vi "Remove Subscriber by Name.vi"(8 "error in (no error)":errorcluster, 10 "Topic Name":string, 11 "Subscriber Look Up Table in":refnum<class "Subscriber Look Up Table.lvclass">) -> (0 "error out":errorcluster, 2 "Found?":bool, 3 "Subscriber Look Up Table out":refnum<class "Subscriber Look Up Table.lvclass">)   [LabVIEW 2016, in "Stream Mediator.lvlib" / "Subscriber Look Up Table.lvclass"]
doc: "--\nCopyright © 2017 Composed SystemsI All rights reserved.\n\nAuthor: Jon McBee <jon.mcbee@composed.io>\n\nThis library is provided \"AS IS\" ,WITHOUT WARRANTIES OR\nCONDITIONS OF ANY KIND, either express or implied.\n\nComposed Systems -- composed.io\n\nStream 0.0.1.1\nJon McBee - Composed Systems\nCopyright (c) 2017, Composed Systems"
uses:
  <userlib>/Composed Systems/Stream/Mediator/Classes/Subscriber Look Up Table/Subscriber Look Up Table.lvclass
  C:/Program Files (x86)/National Instruments/LabVIEW 2016/user.lib/Composed Systems/Stream/Look Up Table/Look Up Table/Look Up Table.lvclass
  <userlib>/Composed Systems/Stream/Look Up Table/Look Up Table/Look Up Table.lvclass
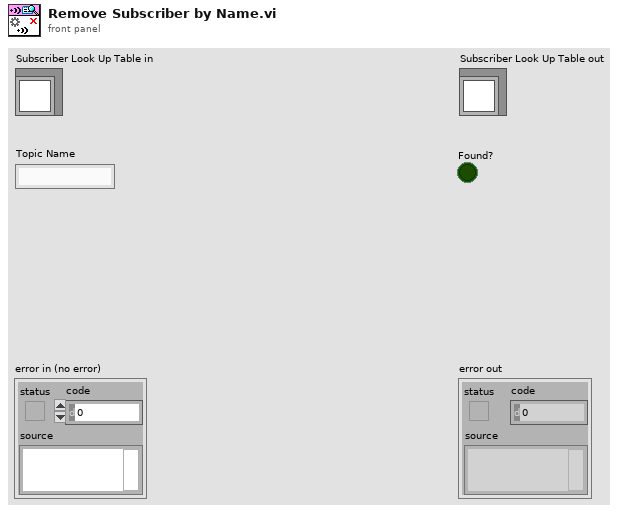
[diagram p1: front panel]
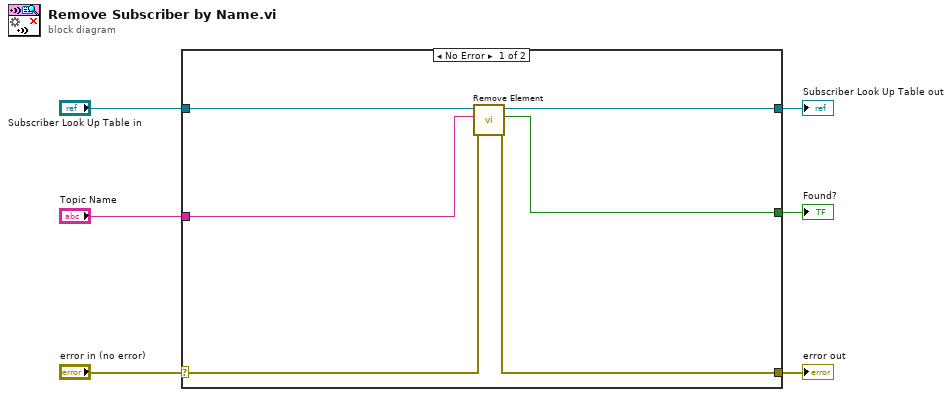
[diagram p0: block diagram]
diagram:
  n1 = case shown="No Error" "error in (no error)" {
    selector: "error in (no error)" -> [w8 w14]
    tunnel: [w7 w14] -> w5
    tunnel: [w11 w13] -> w3
    tunnel: "Subscriber Look Up Table in" -> [w12 w13]
    tunnel: "Topic Name" -> [w10 _]
    tunnel: [w9 _] -> w1
    frame No Error {
      n2 = call <userlib>:"Remove Element.vi"("error in (no error)"=w8, "Name"=w10, "Look Up Table in"=w12) -> ("error out"=w7:errorcluster, "Found?"=w9:bool, "Look Up Table out"=w11:refnum<class "Subscriber Look Up Table.lvclass">)  [unwired: 6 in]
    }
    frame Error {
    }
  }
  "error out" <- w5
  "Subscriber Look Up Table out" <- w3
  "Found?" <- w1
